vi "GetTerminalUID.vi"(6 "error in":errorcluster, 9 "Tunnel in":refnum<class "FlatSequenceInnerTunnel.lvclass">) -> (0 "error out":errorcluster, 3 "Tunnel out":refnum<class "FlatSequenceInnerTunnel.lvclass">, 4 "right terminal UID":i32, 5 "left terminal UID":i32)   [LabVIEW 2014, in "FlatSequenceInnerTunnel.lvclass"]
uses:
  FlatSequenceInnerTunnel.lvclass
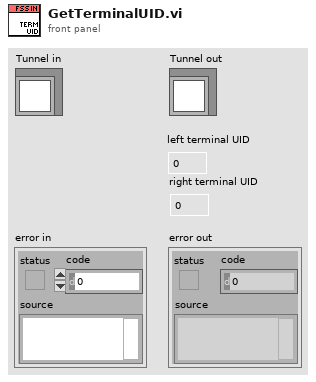
[diagram p1: front panel]
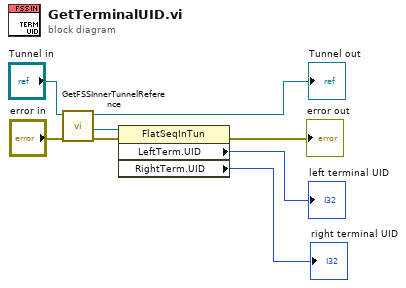
[diagram p0: block diagram]
diagram:
  n1 = call "GetFSSInnerTunnelReference.vi"("error in"="error in", "Tunnel in"="Tunnel in") -> ("error out"=w8:errorcluster, "reference out"=w7:refnum<vi>, "Tunnel out"=→"Tunnel out":refnum<class "FlatSequenceInnerTunnel.lvclass">)  [unwired: 7 in]
  n2 = property class="FlatSeqInTun"(reference=w7, error in=w8) -> (error out=→"error out":errorcluster, "LeftTerm.UID"=→"left terminal UID":i32, "RightTerm.UID"=→"right terminal UID":i32)  [unwired: 1 out]
